vi "encodeNIL.vi"(8 "error in (no error)":errorcluster) -> (0 "error out":errorcluster, 2 "Array":u8[](array[numeric]) format="%.0x")   [LabVIEW 2016, in "MsgPack.lvlib"]
uses:
  MsgPack.lvlib
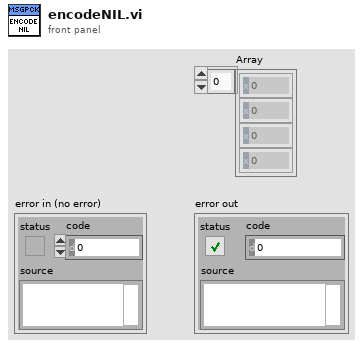
[diagram p1: front panel]
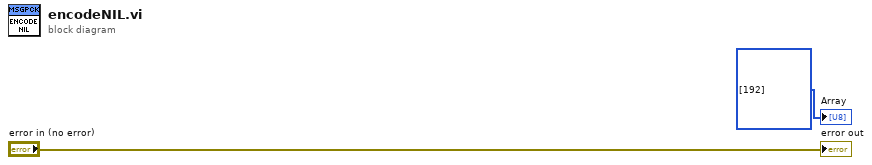
[diagram p0: block diagram]
diagram:
  "Array" <- u8[] [192] ("Array")
  "error out" <- "error in (no error)"
